vi "Xi_for_spline.vi"(1 "Array":dbl[][](array[numeric])) -> (0 "Xi":dbl[](array[numeric]))   [LabVIEW 2015]
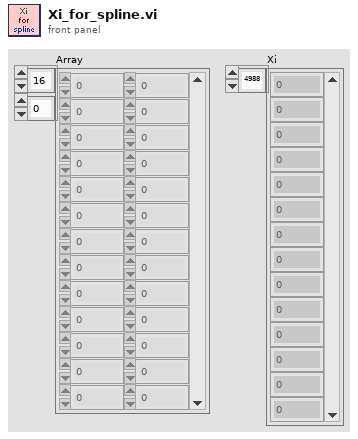
[diagram p1: front panel]
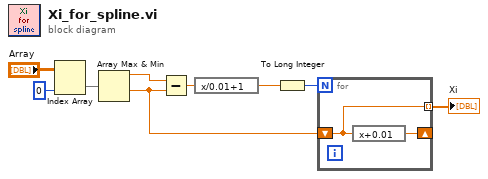
[diagram p0: block diagram]
diagram:
  n1 = Index Array(array="Array", index (col)=0 ("disabled index (col)")) -> (element=w8:dbl[])  [unwired: 1 in]
  n2 = Array Max & Min(array=w8) -> (max value=w7:dbl, min value=w3:dbl)  [unwired: 2 out]
  n3 = Subtract(x=w7, y=w3) -> (x-y=w6:dbl)
  n4 = expression code="x/0.01+1"(w6) -> (w5:dbl)
  n5 = To Long Integer(number=w5) -> (32bit integer=w4:i32)
  n6 = for {
    N: w4 -> [_]
    shift-right: [w11] -> _
    shift-left: w3 -> [w10]
    tunnel: [w10] -> w2 mode=indexing
    n7 = expression code="x+0.01"(w10) -> (w11:dbl)
  }
  "Xi" <- w2
